vi "TestTree.vi"() -> ()   [LabVIEW 2017, in "Client.lvlib" / "UI_API.lvlib"]
uses:
  UI_API.lvlib
  ParserSorter/TypeDefs/SRFields.ctl
  TypeDefs/UIReferences.ctl
  ParserSorter/ParserSorter.lvlib
panel:
  in  "Assigned Sorted SRs":string(tree)
  out "Array 2":string[](array[string])
  out "String":string
  in  "Fields to include":T1[](array[typedef])=[enum."SR Number", enum."Prio", enum."SR Type", enum."Summary", enum."Organisation Name", enum."Days Open"]
  out "data string":string
  out "Array":i32[](array[numeric])
  in  "AE Groups":i32[](listbox)=[0, 1, 2, 3, 4, 5, 6, 7]
  in  "AE Level":enum16{"AE / ELP", "AE Intern"}(ring)
  in  "Tree 2":string(tree)
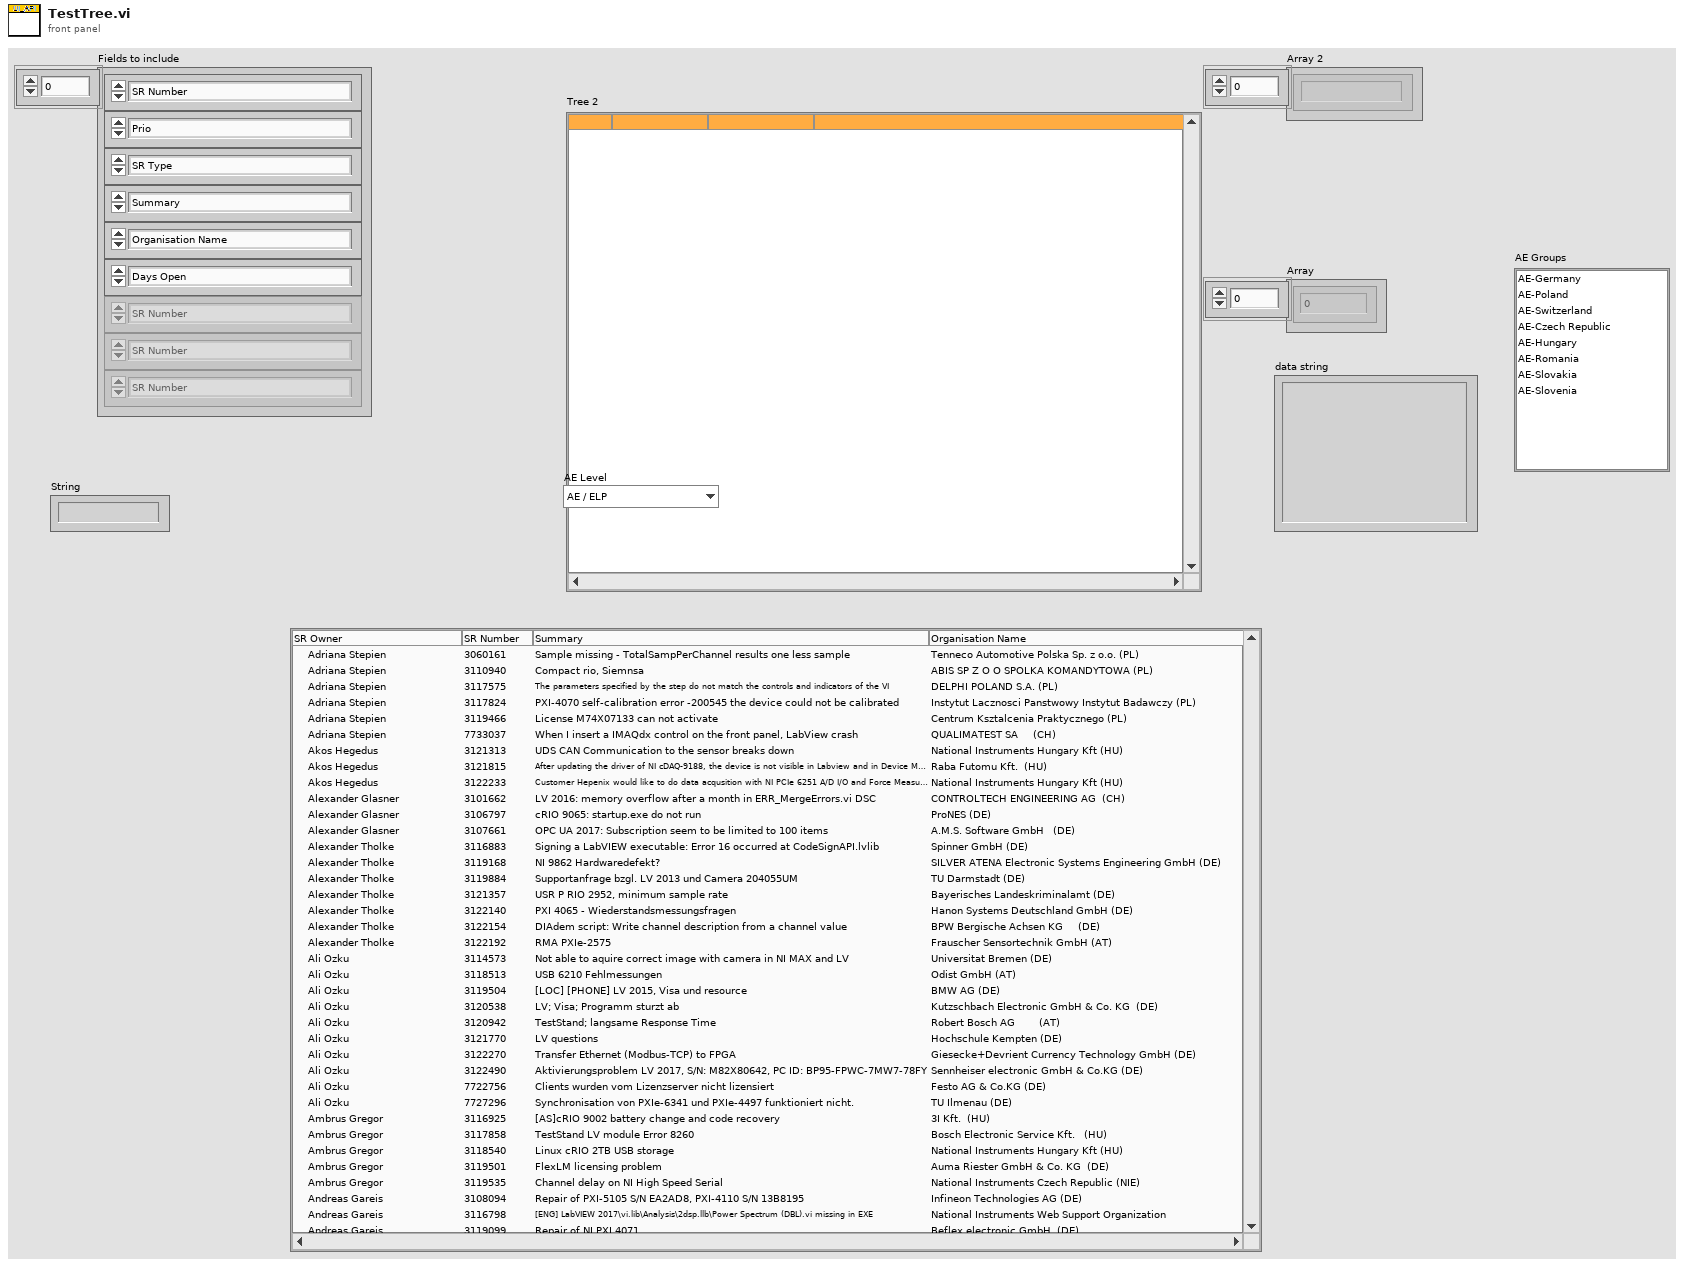
[diagram p1: front panel]
types:
  T1 = typedef "Client.lvlib/ParserSorter.lvlib/SRFields.ctl" = enum16{"SR Number", "AE Group", "SR Owner", "Summary", "SR Status", "Days Open", "Prio", "SR Type", "Service Level", "Last Updated", "First Name", "Last Name", "Organisation Name", "Creation Date", "Needs Merging?", "English Flag?"}
  T2 = typedef "Client.lvlib/UI_API.lvlib/UIReferences.ctl" = cluster{"Assigned SRs":refnum<vi>, "Unassigned SRs":refnum<vi>, "AE Level":refnum<vi>, "AE Groups":refnum<vi>}
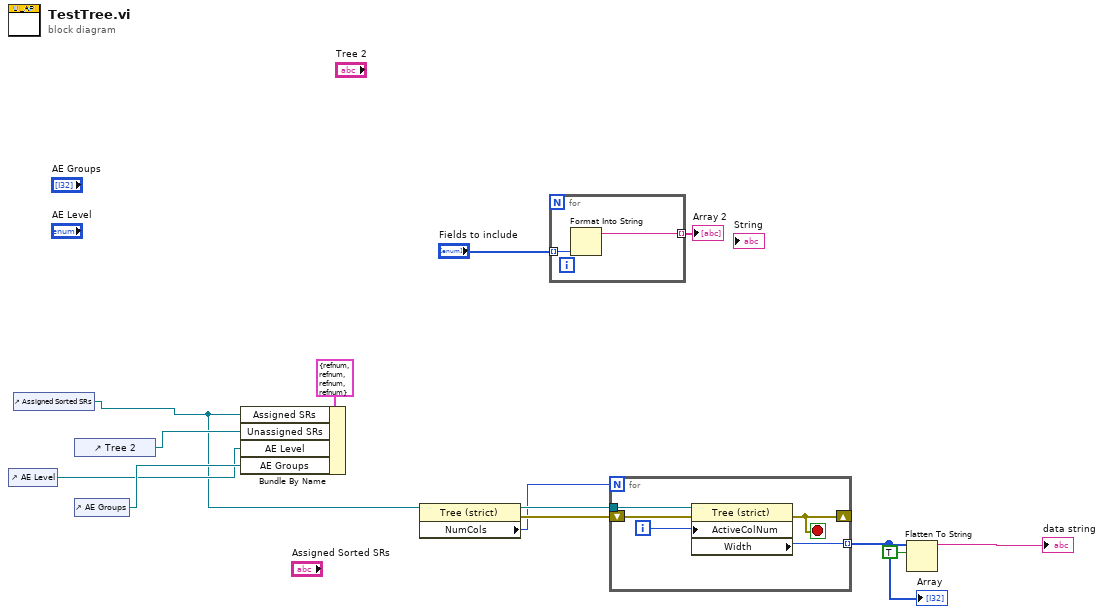
[diagram p0: block diagram]
diagram:
  n1 = control-ref of="AE Level"() -> (w10:refnum<vi>)
  n2 = control-ref of="Assigned Sorted SRs"() -> (w1:refnum<vi>)
  n3 = control-ref of="Tree 2"() -> (w12:refnum<vi>)
  n4 = control-ref of="AE Groups"() -> (w11:refnum<vi>)
  n5 = Bundle By Name(cluster=T2 {"Assigned SRs"=refnum, "Unassigned SRs"=refnum, "AE Level"=refnum, "AE Groups"=refnum} ("UI References"), "Assigned SRs"=w1, "Unassigned SRs"=w12, "AE Level"=w10, "AE Groups"=w11) -> ()  [unwired: 1 out]
  n6 = property class="Tree (strict)"(reference=w1) -> (reference out=w8:refnum<vi>, error out=w9:errorcluster, "NumCols"=w5:u32)  [unwired: 1 in]
  n7 = for {
    tunnel: "Fields to include" -> [w15] mode=indexing
    tunnel: [w14] -> w2 mode=indexing
    n8 = Format Into String(w15) -> (resulting string=w14:string)  [unwired: 3 in, 1 out]
  }
  "Array 2" <- w2
  n9 = for {
    N: w5 -> [_]
    shift-right: [w19] -> _
    shift-left: w9 -> [w20]
    tunnel: [w17] -> w7 mode=indexing
    tunnel: w8 -> [w16]
    i -> [w18]
    stop <- w19 stop-if-true
    n10 = property class="Tree (strict)"(reference=w16, error in=w20, "ActiveColNum"=w18) -> (error out=w19:errorcluster, "Width"=w17:i32)  [unwired: 1 out]
  }
  "Array" <- w7
  n11 = Flatten To String(anything=w7, prepend array or string size? (T)=TRUE) -> (data string=→"data string":string)  [unwired: 2 in, 2 out]
